vi "Read Actual Position_all.vi"(4 "error in (no error)":errorcluster, 5 "ESP302":refnum<class "ESP302.lvclass">, 7 "VISA resource name":refnum<visa-resource-name>) -> (0 "error out":errorcluster, 1 "ESP302 out":refnum<class "ESP302.lvclass">, 2 "positions":dbl[](array[numeric]), 3 "VISA resource name out":refnum<visa-resource-name>)   [LabVIEW 2020, in "ESP302.lvclass"]
doc: "Reads the current position.\nIt returns the instantaneous real position of the specified axis."
uses:
  ESP302.lvclass
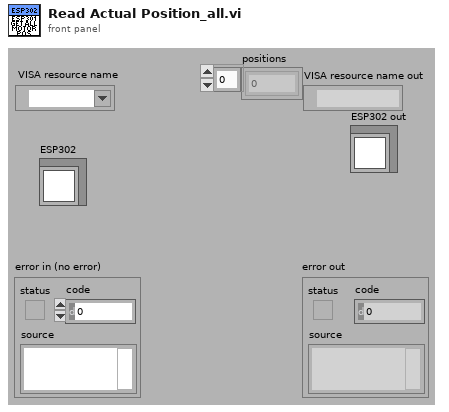
[diagram p1: front panel]
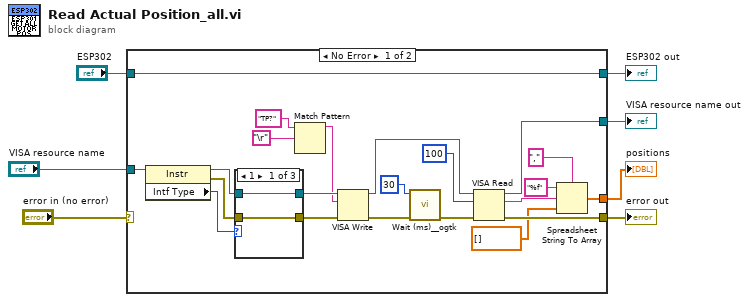
[diagram p0: block diagram]
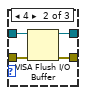
[diagram p2: hidden frame]
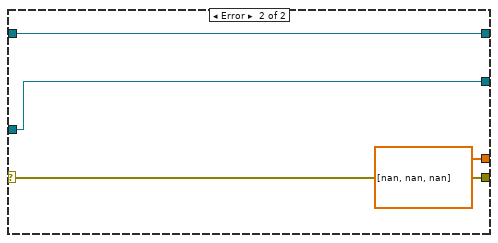
[diagram p4: hidden frame]
diagram:
  n1 = case shown="No Error" "error in (no error)" {
    selector: "error in (no error)" -> [_ w39]
    tunnel: "VISA resource name" -> [w18 w40]
    tunnel: [w17 w39] -> w6
    tunnel: [w16 w40] -> w5
    tunnel: "ESP302" -> [w15 w41]
    tunnel: [w15 w41] -> w2
    tunnel: [w14 dbl[] [nan, nan, nan]] -> w1
    frame No Error {
      n2 = property class="Instr"(reference=w18) -> (reference out=w23:refnum<visa-resource-name>, error out=w22:errorcluster, "Intf Type"=w24:u16)  [unwired: 1 in]
      n3 = case shown="1" w24 {
        tunnel: w23 -> [w31 w33 w37]
        tunnel: [w31 w32 w37] -> w28
        tunnel: w22 -> [w30 w35 w36]
        tunnel: [w30 w34 w36] -> w27
        frame 1 {
        }
        frame 4 {
          n4 = VISA Flush I/O Buffer(VISA resource name=w33, error in (no error)=w35) -> (VISA resource name out=w32:refnum<visa-resource-name>, error out=w34:errorcluster)  [unwired: 1 out]
        }
        frame Default {
        }
      }
      n5 = Match Pattern(string="TP?" ("Read Actual\nPosition"), regular expression="\r") -> (before substring=w20:string)  [unwired: 4 out]
      n6 = VISA Write(VISA resource name=w28, write buffer=w20, error in (no error)=w27) -> (VISA resource name out=w29:refnum<visa-resource-name>, error out=w26:errorcluster)  [unwired: 1 out]
      n7 = call <userlib>:"Wait (ms)__ogtk.vi"("error in (no error)"=w26, "milliseconds to wait"=u32 30 ("Wait before read (0ms)")) -> ("error out"=w13:errorcluster)  [unwired: 8 in, 1 out]
      n8 = VISA Read(VISA resource name=w29, byte count=u32 100 ("Bytes to read (100)"), error in (no error)=w13) -> (VISA resource name out=w16:refnum<visa-resource-name>, read buffer=w11:string, error out=w17:errorcluster)  [unwired: 1 out]
      n9 = Spreadsheet String To Array(delimiter (Tab)=",", format string="%f", spreadsheet string=w11, array type (2D Dbl)=dbl[] []) -> (array=w14:dbl[])
    }
    frame Error {
    }
  }
  "error out" <- w6
  "VISA resource name out" <- w5
  "ESP302 out" <- w2
  "positions" <- w1
